vi "Translator C Basic Lib.vi"(0 "Input":variant=variant("Function Name"=variant(string "Strip Path"), "Input Datatypes"=variant(string[] ["error", "int"]), "Inputs"=variant(string[] ["error in", "x"]), "Node refnum"=variant(refnum<vi> refnum), "Output Datatypes"=variant(string[] ["int"]), "Outputs"=variant(string[] ["a"])), 11 "error in (no error)":errorcluster) -> (4 "Output":variant=variant("Defines"=variant(string[] []), "Includes"=variant(string[] []), "Replaced Code"=variant(string "/* LabVIEW system function 'Strip Path' not found. */")), 15 "error out":errorcluster)   [LabVIEW 2014, in "C Basic Lib.lvlib"]
doc: "source: https://www.arduino.cc/en/Reference/SPIEnd\n\nDisables the SPI bus (leaving pin modes unchanged).\n\nSyntax\n SPI.end()\n\nParameters\n None\n\nReturns\n None"
uses:
  C Basic Lib.lvlib
panel:
  out "Outputs":string[](array[string])
  out "Inputs":string[](array[string])
  out "Output Datatypes":string[](array[string])
  out "Input Datatypes":string[](array[string])
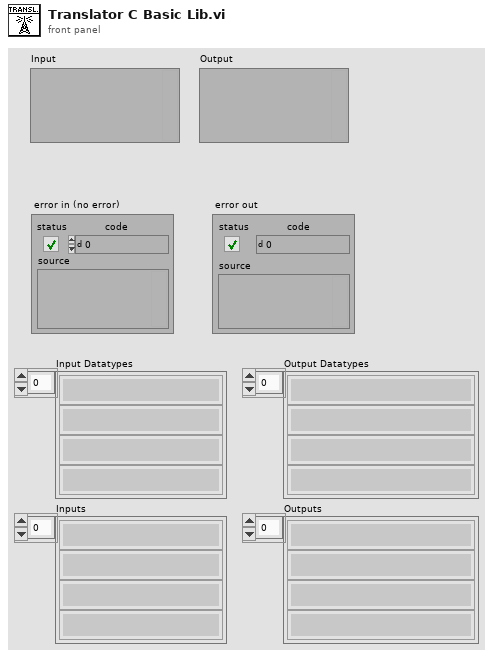
[diagram p1: front panel]
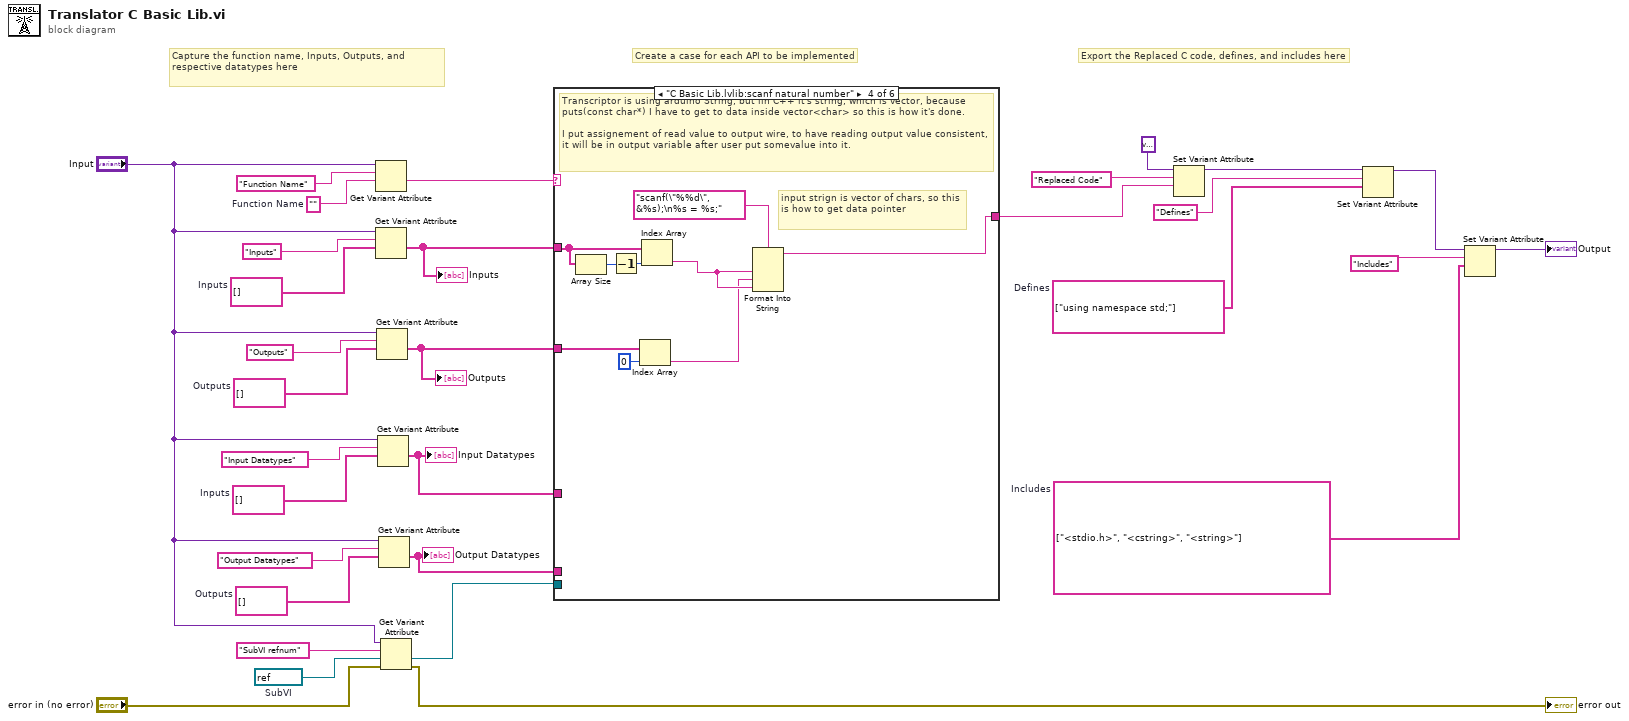
[diagram p0: block diagram]
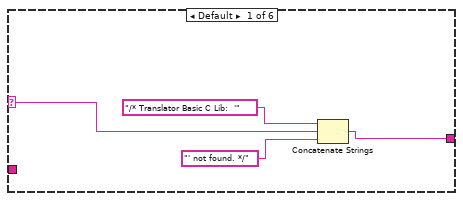
[diagram p2: hidden frame]
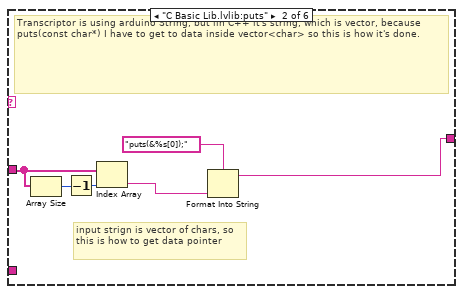
[diagram p3: hidden frame]
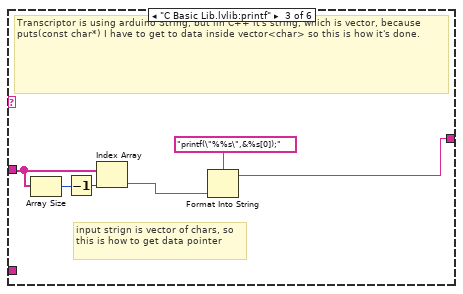
[diagram p4: hidden frame]
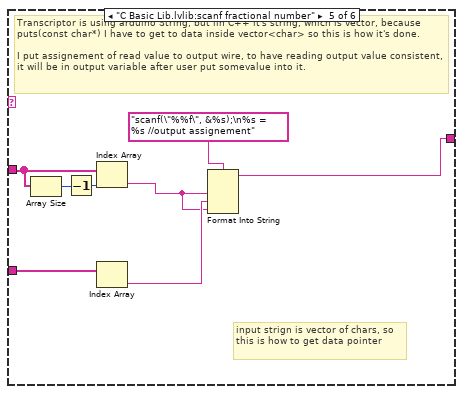
[diagram p5: hidden frame]
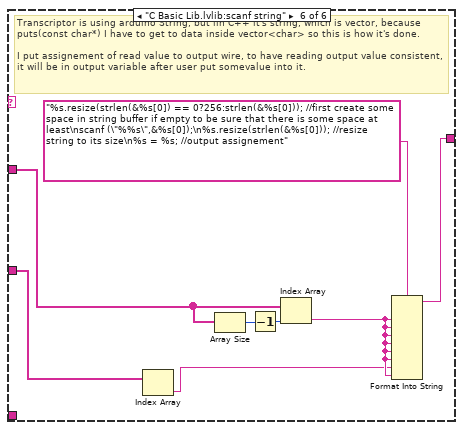
[diagram p6: hidden frame]
diagram:
  w7 = refnum<vi> refnum  # SubVI
  w4 = string[] ["using namespace std;"]  # Defines
  w17 = string[] []  # Outputs
  w18 = string[] []  # Inputs
  w3 = string[] ["<stdio.h>", "<cstring>", "<string>"]  # Includes
  w27 = string[] []  # Outputs
  w28 = string[] []  # Inputs
  w29 = ""  # Function Name
  # "Capture the function name, Inputs, Outputs, and respective datatypes here"
  # "Export the Replaced C code, defines, and includes here"
  # "Create a case for each API to be implemented"
  n1 = Get Variant Attribute(Variant="Input", name="Function Name", default value (empty Variant)=w29) -> (value=w24:string)  [unwired: 1 in, 3 out]
  n2 = Get Variant Attribute(Variant="Input", name="Inputs", default value (empty Variant)=w28) -> (value=w14:string[])  [unwired: 1 in, 3 out]
  "Inputs" <- w14
  n3 = Get Variant Attribute(Variant="Input", name="Outputs", default value (empty Variant)=w27) -> (value=w15:string[])  [unwired: 1 in, 3 out]
  "Outputs" <- w15
  n4 = Get Variant Attribute(Variant="Input", name="Input Datatypes", default value (empty Variant)=w18) -> (value=w10:string[])  [unwired: 1 in, 3 out]
  "Input Datatypes" <- w10
  n5 = Get Variant Attribute(Variant="Input", name="Output Datatypes", default value (empty Variant)=w17) -> (value=w5:string[])  [unwired: 1 in, 3 out]
  "Output Datatypes" <- w5
  n6 = Get Variant Attribute(Variant="Input", name="SubVI refnum", default value (empty Variant)=w7, error in="error in (no error)") -> (value=w6:refnum<vi>, error out=→"error out":errorcluster)  [unwired: 2 out]
  n7 = case shown="\"C Basic Lib.lvlib:scanf natural number\"" w24 {
    selector: w24 -> [w34 _ _ _ _ _]
    tunnel: [w32 w39 w45 w55 w63 w72] -> w23
    tunnel: w14 -> [_ w38 w44 w54 w62 w69]
    tunnel: w15 -> [_ _ _ w50 w59 w66]
    tunnel: w10 -> [_ _ _ _ _ _]
    tunnel: w6 -> [_ _ _ _ _ _]
    tunnel: w5 -> [_ _ _ _ _ _]
    frame Default {
      n8 = Concatenate Strings("/* Translator Basic C Lib:  '", w34, "' not found. */") -> (w32:string)
    }
    frame "C Basic Lib.lvlib:puts" {
      # "input strign is vector of chars, so this is how to get data pointer"
      # "Transcriptor is using arduino String, but iin C++ it's string, which is vector, because puts(const char*) I have to get to data inside vector<char> so this is how it's done."
      n9 = Array Size(array=w38) -> (size(s)=w37:i32)
      n10 = Decrement(x=w37) -> (x-1=w36:i32)
      n11 = Index Array(array=w38, index=w36) -> (element=w40:string)
      n12 = Format Into String(format string="puts(&%s[0]);", w40) -> (resulting string=w39:string)  [unwired: 2 in, 1 out]
    }
    frame "C Basic Lib.lvlib:printf" {
      # "input strign is vector of chars, so this is how to get data pointer"
      # "Transcriptor is using arduino String, but iin C++ it's string, which is vector, because puts(const char*) I have to get to data inside vector<char> so this is how it's done."
      n13 = Array Size(array=w44) -> (size(s)=w43:i32)
      n14 = Decrement(x=w43) -> (x-1=w42:i32)
      n15 = Index Array(array=w44, index=w42) -> (element=w46:string)
      n16 = Format Into String(format string="printf(\"%%s\",&%s[0]);", w46) -> (resulting string=w45:string)  [unwired: 2 in, 1 out]
    }
    frame "C Basic Lib.lvlib:scanf natural number" {
      # "input strign is vector of chars, so this is how to get data pointer"
      # "Transcriptor is using arduino String, but iin C++ it's string, which is vector, because puts(const char*) I have to get to data inside vector<char> so this is how it's done.\n\nI put assignement of read value to output wire, to have reading output value consistent, it will be in output variable after user put somevalue into it."
      n17 = Array Size(array=w54) -> (size(s)=w53:i32)
      n18 = Decrement(x=w53) -> (x-1=w52:i32)
      n19 = Index Array(array=w50, index=0) -> (element=w49:string)
      n20 = Index Array(array=w54, index=w52) -> (element=w51:string)
      n21 = Format Into String(format string="scanf(\"%%d\", &%s);\n%s = %s;", w51, w49, w51) -> (resulting string=w55:string)  [unwired: 2 in, 1 out]
    }
    frame "C Basic Lib.lvlib:scanf fractional number" {
      # "input strign is vector of chars, so this is how to get data pointer"
      # "Transcriptor is using arduino String, but iin C++ it's string, which is vector, because puts(const char*) I have to get to data inside vector<char> so this is how it's done.\n\nI put assignement of read value to output wire, to have reading output value consistent, it will be in output variable after user put somevalue into it."
      n22 = Array Size(array=w62) -> (size(s)=w61:i32)
      n23 = Decrement(x=w61) -> (x-1=w60:i32)
      n24 = Index Array(array=w62, index=w60) -> (element=w57:string)
      n25 = Index Array(array=w59) -> (element=w58:string)  [unwired: 1 in]
      n26 = Format Into String(format string="scanf(\"%%f\", &%s);\n%s = %s //output assignement", w57, w58, w57) -> (resulting string=w63:string)  [unwired: 2 in, 1 out]
    }
    frame "C Basic Lib.lvlib:scanf string" {
      # "Transcriptor is using arduino String, but iin C++ it's string, which is vector, because puts(const char*) I have to get to data inside vector<char> so this is how it's done.\n\nI put assignement of read value to output wire, to have reading output value consistent, it will be in output variable after user put somevalue into it."
      n27 = Index Array(array=w66) -> (element=w65:string)  [unwired: 1 in]
      n28 = Array Size(array=w69) -> (size(s)=w71:i32)
      n29 = Decrement(x=w71) -> (x-1=w70:i32)
      n30 = Index Array(array=w69, index=w70) -> (element=w67:string)
      n31 = Format Into String(format string="%s.resize(strlen(&%s[0]) == 0?256:strlen(&%s[0])); //first create some space in string buffer if empty to be sure that there is some space at least\nscanf (\"%%s\",&%s[0]);\n%s.resize(strlen(&%s[0])); //resize string to its size\n%s = %s; //output assignement", w67, w67, w67, w67, w67, w67, w65, w67) -> (resulting string=w72:string)  [unwired: 2 in, 1 out]
    }
  }
  n32 = Set Variant Attribute(Variant=variant ("variant"), name="Replaced Code", value=w23) -> (Variant out=w13:variant)  [unwired: 1 in, 2 out]
  n33 = Set Variant Attribute(Variant=w13, name="Defines", value=w4) -> (Variant out=w12:variant)  [unwired: 1 in, 2 out]
  n34 = Set Variant Attribute(Variant=w12, name="Includes", value=w3) -> (Variant out=→"Output":variant)  [unwired: 1 in, 2 out]
